vi "DSF.Engine.Execution.Builder.Get FIFOs.vi"(8 "error in (no error)":errorcluster, 11 "Builder in":refnum<class "DSF.Engine.Execution.Builder.lvclass">) -> (0 "error out":errorcluster, 2 "FIFOs":T1, 3 "Builder out":refnum<class "DSF.Engine.Execution.Builder.lvclass">)   [LabVIEW 2016, in "DSF.Engine.lvlib" / "DSF.Engine.Execution.Builder.lvclass"]
uses:
  DSF.Engine.Execution.Builder.lvclass
  DSF.Engine.Execution.Builder.FIFOs.ctl
  DSF.Engine.Execution.Builder.Command FIFO.ctl
  DSF.Engine.Execution.Builder.Command Payload.ctl
  DSF.Engine.Execution.Builder.Commands.ctl
  DSF.Engine.Execution.Builder.Response FIFO.ctl
  DSF.Engine.Execution.Builder.Response Payload.ctl
  DSF.Engine.Execution.Builder.lvclass/DSF.Engine.Execution.Builder.ctl
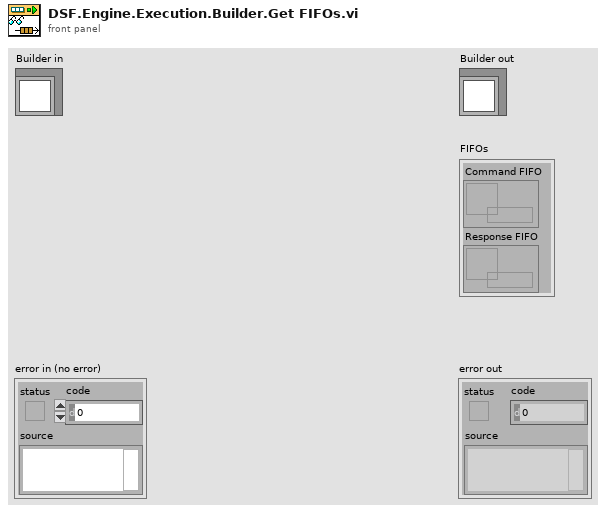
[diagram p1: front panel]
types:
  T1 = typedef "DSF.Engine.lvlib/DSF.Engine.Execution.Builder.lvclass/DSF.Engine.Execution.Builder.FIFOs.ctl" = cluster{"Command FIFO":T2, "Response FIFO":T3}
  T2 = typedef "DSF.Engine.lvlib/DSF.Engine.Execution.Builder.lvclass/DSF.Engine.Execution.Builder.Command FIFO.ctl" = refnum<k33>
  T3 = typedef "DSF.Engine.lvlib/DSF.Engine.Execution.Builder.lvclass/DSF.Engine.Execution.Builder.Response FIFO.ctl" = refnum<k33>
  T4 = typedef "DSF.Engine.lvlib/DSF.Execution.Builder.lvclass/DSF.Engine.Execution.Builder.FIFOs.ctl" = cluster{"Command FIFO":T5, "Response FIFO":T6}
  T5 = typedef "DSF.Engine.lvlib/DSF.Execution.Builder.lvclass/DSF.Engine.Execution.Builder.Command FIFO.ctl" = refnum<k33>
  T6 = typedef "DSF.Engine.lvlib/DSF.Execution.Builder.lvclass/DSF.Engine.Execution.Builder.Response FIFO.ctl" = refnum<k33>
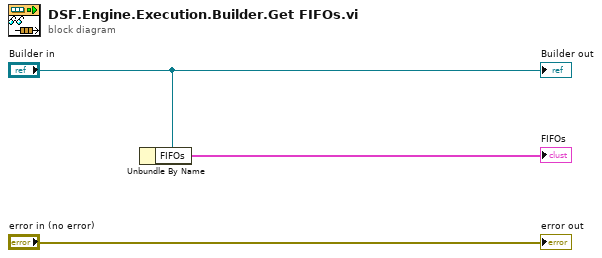
[diagram p0: block diagram]
diagram:
  n1 = Unbundle By Name("Builder in") -> ("FIFOs"=→"FIFOs":T4)
  "error out" <- "error in (no error)"
  "Builder out" <- "Builder in"
